vi "PktHeader - Header Array to Strings.vi"(8 "error in (no error)":errorcluster, 11 "Header Array In":bool[](array[boolean])) -> (0 "error out":errorcluster, 1 "Data Name String":string, 2 "Num Bits String":string, 3 "Header Array Out":bool[](array[boolean]))   [LabVIEW 2019, in "UDP-Custom-Device System Explorer.lvlib"]
uses:
  UDP-Custom-Device System Explorer.lvlib
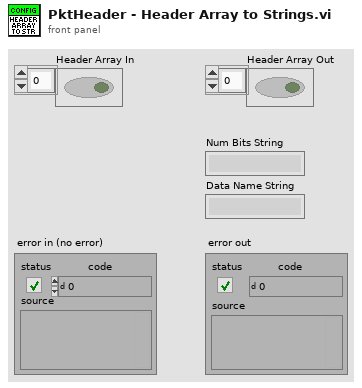
[diagram p1: front panel]
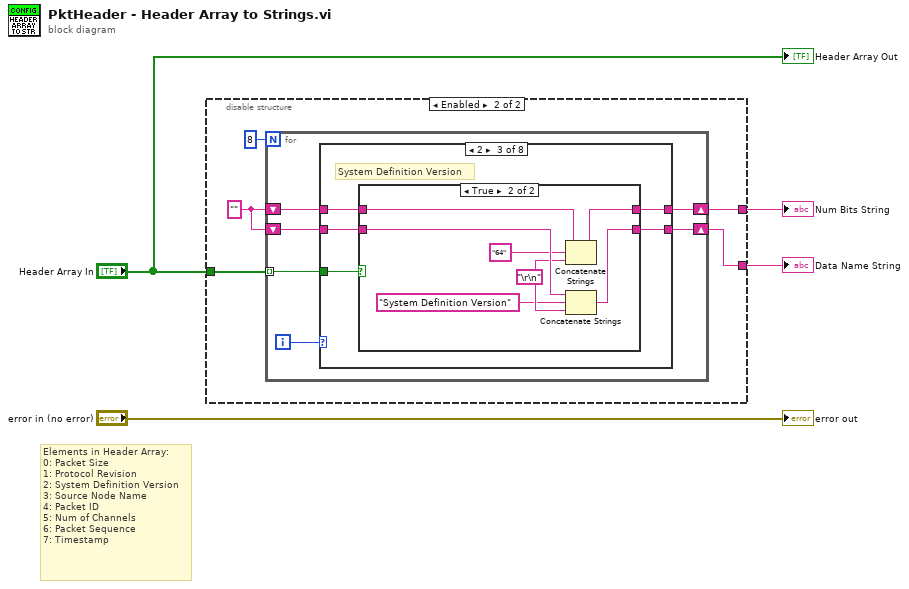
[diagram p0: block diagram]
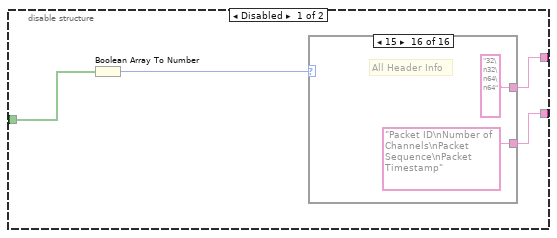
[diagram p2: hidden frame]
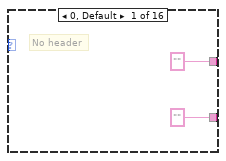
[diagram p3: hidden frame]
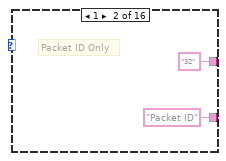
[diagram p4: hidden frame]
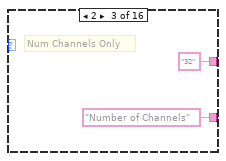
[diagram p5: hidden frame]
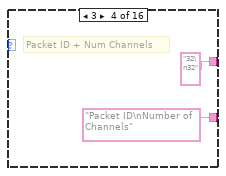
[diagram p6: hidden frame]
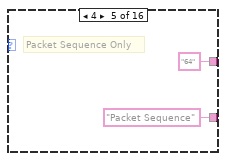
[diagram p7: hidden frame]
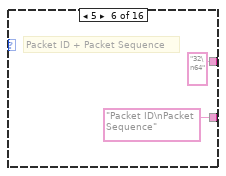
[diagram p8: hidden frame]
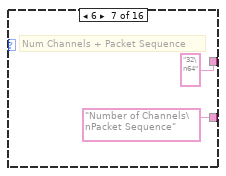
[diagram p9: hidden frame]
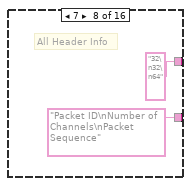
[diagram p10: hidden frame]
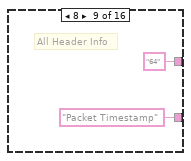
[diagram p11: hidden frame]
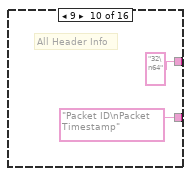
[diagram p12: hidden frame]
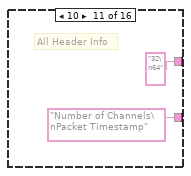
[diagram p13: hidden frame]
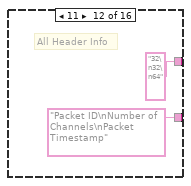
[diagram p14: hidden frame]
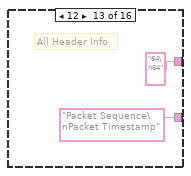
[diagram p15: hidden frame]
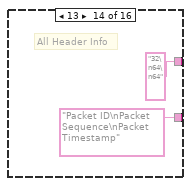
[diagram p16: hidden frame]
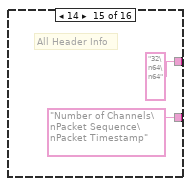
[diagram p17: hidden frame]
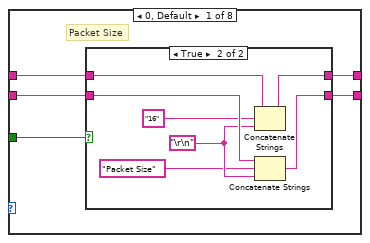
[diagram p18: hidden frame]
diagram:
  # "Elements in Header Array:\n0: Packet Size\n1: Protocol Revision\n2: System Definition Version\n3: Source Node Name\n4: Packet ID\n5: Num of Channels\n6: Packet Sequence\n7: Timestamp"
  n1 = disable-structure shown="Enabled" {
    disable-tunnel: [w7 w43] -> w4
    disable-tunnel: [w6 w42] -> w3
    disable-tunnel: "Header Array In" -> [w5 w44]
    frame Disabled {
      n2 = Boolean Array To Number(Boolean array=w5) -> (number=w8:u32)
      n3 = case shown="15" w8 {
        tunnel: ["" "32" "32" "32\n32" "64" "32\n64" "32\n64" "32\n32\n64" "64" "32\n64" "32\n64" "32\n32\n64" "64\n64" "32\n64\n64" "32\n64\n64" "32\n32\n64\n64"] -> w7
        tunnel: ["" "Packet ID" "Number of Channels" "Packet ID\nNumber of Channels" "Packet Sequence" "Packet ID\nPacket Sequence" "Number of Channels\nPacket Sequence" "Packet ID\nNumber of Channels\nPacket Sequence" "Packet Timestamp" "Packet ID\nPacket Timestamp" "Number of Channels\nPacket Timestamp" "Packet ID\nNumber of Channels\nPacket Timestamp" "Packet Sequence\nPacket Timestamp" "Packet ID\nPacket Sequence\nPacket Timestamp" "Number of Channels\nPacket Sequence\nPacket Timestamp" "Packet ID\nNumber of Channels\nPacket Sequence\nPacket Timestamp"] -> w6
        frame 0, Default {
          # "No header"
        }
        frame 1 {
          # "Packet ID Only"
        }
        frame 2 {
          # "Num Channels Only"
        }
        frame 3 {
          # "Packet ID + Num Channels"
        }
        frame 4 {
          # "Packet Sequence Only"
        }
        frame 5 {
          # "Packet ID + Packet Sequence"
        }
        frame 6 {
          # "Num Channels + Packet Sequence"
        }
        frame 7 {
          # "All Header Info"
        }
        frame 8 {
          # "All Header Info"
        }
        frame 9 {
          # "All Header Info"
        }
        frame 10 {
          # "All Header Info"
        }
        frame 11 {
          # "All Header Info"
        }
        frame 12 {
          # "All Header Info"
        }
        frame 13 {
          # "All Header Info"
        }
        frame 14 {
          # "All Header Info"
        }
        frame 15 {
          # "All Header Info"
        }
      }
    }
    frame Enabled {
      w45 = ""
      n4 = for {
        N: 8 -> [_]
        shift-right: [w49] -> w43
        shift-left: w45 -> [w48]
        shift-right: [w47] -> w42
        shift-left: w45 -> [w46]
        tunnel: w44 -> [w50] mode=indexing
        i -> [w51]
        n5 = case shown="2" w51 {
          tunnel: w50 -> [w52 w66 w80 w94 w108 w122 w136 w150]
          tunnel: [w55 w69 w83 w97 w111 w125 w139 w153] -> w49
          tunnel: w48 -> [w56 w70 w84 w98 w112 w126 w140 w154]
          tunnel: [w53 w67 w81 w95 w109 w123 w137 w151] -> w47
          tunnel: w46 -> [w54 w68 w82 w96 w110 w124 w138 w152]
          frame 0, Default {
            # "Packet Size"
            n6 = case shown="True" w52 {
              tunnel: w56 -> [w58 w65]
              tunnel: [w58 w64] -> w55
              tunnel: w54 -> [w57 w63]
              tunnel: [w57 w62] -> w53
              frame False {
              }
              frame True {
                w60 = "\r\n"
                n7 = Concatenate Strings(w65, "16" ("string"), w60) -> (w64:string)
                n8 = Concatenate Strings(w63, "Packet Size" ("string"), w60) -> (w62:string)
              }
            }
          }
          frame 1 {
            # "Protocol Revision"
            n9 = case shown="False" w66 {
              tunnel: w70 -> [w72 w79]
              tunnel: [w72 w78] -> w69
              tunnel: w68 -> [w71 w77]
              tunnel: [w71 w76] -> w67
              frame False {
              }
              frame True {
                w74 = "\r\n"
                n10 = Concatenate Strings(w79, "8" ("string"), w74) -> (w78:string)
                n11 = Concatenate Strings(w77, "Protocol Revision" ("string"), w74) -> (w76:string)
              }
            }
          }
          frame 2 {
            # "System Definition Version"
            n12 = case shown="True" w80 {
              tunnel: w84 -> [w86 w93]
              tunnel: [w86 w92] -> w83
              tunnel: w82 -> [w85 w91]
              tunnel: [w85 w90] -> w81
              frame False {
              }
              frame True {
                w88 = "\r\n"
                n13 = Concatenate Strings(w93, "64" ("string"), w88) -> (w92:string)
                n14 = Concatenate Strings(w91, "System Definition Version" ("string"), w88) -> (w90:string)
              }
            }
          }
          frame 3 {
            # "Source Node Name"
            n15 = case shown="True" w94 {
              tunnel: w98 -> [w100 w107]
              tunnel: [w100 w106] -> w97
              tunnel: w96 -> [w99 w105]
              tunnel: [w99 w104] -> w95
              frame False {
              }
              frame True {
                w102 = "\r\n"
                n16 = Concatenate Strings(w107, "256" ("string"), w102) -> (w106:string)
                n17 = Concatenate Strings(w105, "Source Node Name" ("string"), w102) -> (w104:string)
              }
            }
          }
          frame 4 {
            # "Packet ID"
            n18 = case shown="True" w108 {
              tunnel: w112 -> [w114 w121]
              tunnel: [w114 w120] -> w111
              tunnel: w110 -> [w113 w119]
              tunnel: [w113 w118] -> w109
              frame False {
              }
              frame True {
                w116 = "\r\n"
                n19 = Concatenate Strings(w121, "32" ("string"), w116) -> (w120:string)
                n20 = Concatenate Strings(w119, "Packet ID" ("string"), w116) -> (w118:string)
              }
            }
          }
          frame 5 {
            # "Num of Channels"
            n21 = case shown="True" w122 {
              tunnel: w126 -> [w128 w135]
              tunnel: [w128 w134] -> w125
              tunnel: w124 -> [w127 w133]
              tunnel: [w127 w132] -> w123
              frame False {
              }
              frame True {
                w130 = "\r\n"
                n22 = Concatenate Strings(w135, "32" ("string"), w130) -> (w134:string)
                n23 = Concatenate Strings(w133, "Channel Count" ("string"), w130) -> (w132:string)
              }
            }
          }
          frame 6 {
            # "Packet Sequence"
            n24 = case shown="True" w136 {
              tunnel: w140 -> [w142 w149]
              tunnel: [w142 w148] -> w139
              tunnel: w138 -> [w141 w147]
              tunnel: [w141 w146] -> w137
              frame False {
              }
              frame True {
                w144 = "\r\n"
                n25 = Concatenate Strings(w149, "64" ("string"), w144) -> (w148:string)
                n26 = Concatenate Strings(w147, "Packet Sequence" ("string"), w144) -> (w146:string)
              }
            }
          }
          frame 7 {
            # "Timestamp"
            n27 = case shown="True" w150 {
              tunnel: w154 -> [w156 w163]
              tunnel: [w156 w162] -> w153
              tunnel: w152 -> [w155 w161]
              tunnel: [w155 w160] -> w151
              frame False {
              }
              frame True {
                w158 = "\r\n"
                n28 = Concatenate Strings(w163, "64" ("string"), w158) -> (w162:string)
                n29 = Concatenate Strings(w161, "Timestamp" ("string"), w158) -> (w160:string)
              }
            }
          }
        }
      }
    }
  }
  "Num Bits String" <- w4
  "Data Name String" <- w3
  "Header Array Out" <- "Header Array In"
  "error out" <- "error in (no error)"
